vi "Arduino Drive.vi"() -> ()   [LabVIEW 2013]
panel:
  out "Back Flower Activated?":bool
  out "Right Flower Activated?":bool
  out "Intake Activated?":bool
  out "Intake -1, 1 (Suck In/Suck Out)":dbl
  out "Doggear Out/Engaged (T/F)":bool
  out "Back Flower Out/In (T/F)":bool
  out "Right Flower Out/In (T/F)":bool
  out "Intake Out/In (T/F)":bool
  in  "KeyInput":T1(ring)
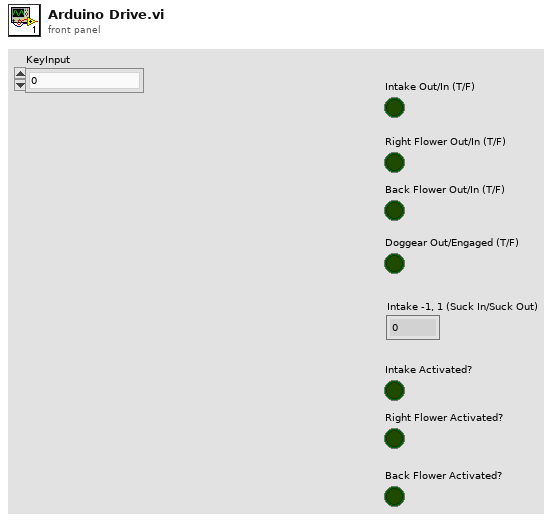
[diagram p1: front panel]
types:
  T1 = enum16{"0", "1", "2", "3", "4", "5", "6", "7", "8", "9", "A", "B", "C", "D", "E", "F", "G", "H", "I", "J", "K", "L", "M", "N", "O", "P", "Q", "R", "S", "T", "U", "V", "W", "X", "Y", "Z", "F1", "F2", "F3", "F4", "F5", "F6", "F7", "F8", "F9", "F10", "F11", "F12", "F13", "F14", "F15", "ADD", "BACK", "BACKSLASH", "CAPITAL", "COMMA", "DECIMAL", "DELETE", "DIVIDE", "DOWN", "END", "EQUALS", "ESCAPE", "GRAVE (`)", "HOME", "INSERT", "LBRACKET", "LCONTROL", "LEFT", "L ALT", "LSHIFT", "LWIN", "MINUS", "MULTIPLY", "NEXT", "NUMLOCK", "NUMPAD_0", "NUMPAD_1", "NUMPAD_2", "NUMPAD_3", "NUMPAD_4", "NUMPAD_5", "NUMPAD_6", "NUMPAD_7", "NUMPAD_8", "NUMPAD_9", "PAUSE", "PERIOD", "PRIOR (PG UP)", "RBRACKET", "RCONTROL", "RETURN", "RIGHT", "R ALT", "RSHIFT", "RWIN", "SCROLL", "SEMICOLON", "SLASH", "SPACE", "SUBTRACT", "TAB", "UP", "ENTER (num pad)", "' (quote)"}
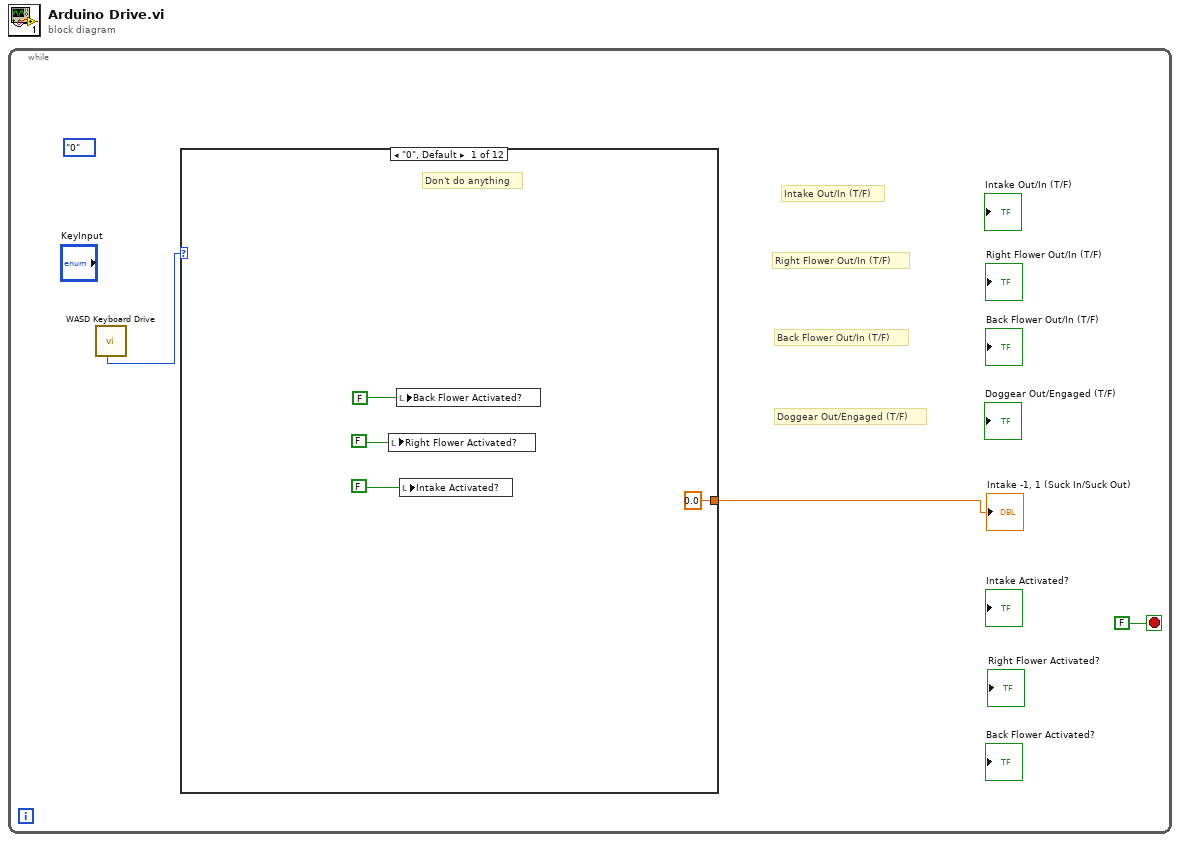
[diagram p0: block diagram]
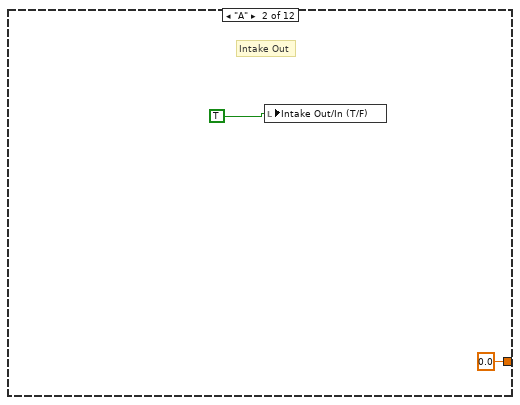
[diagram p2: hidden frame]
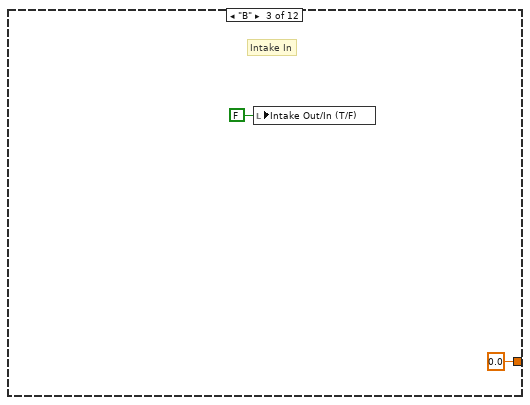
[diagram p3: hidden frame]
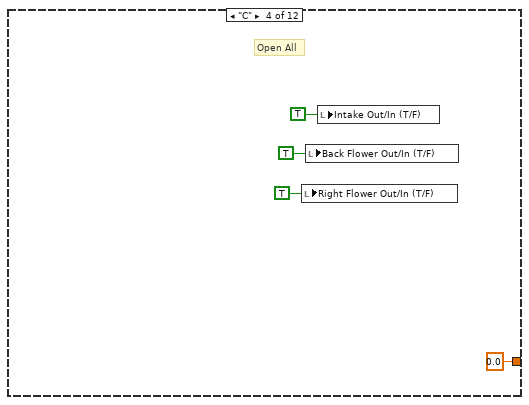
[diagram p4: hidden frame]
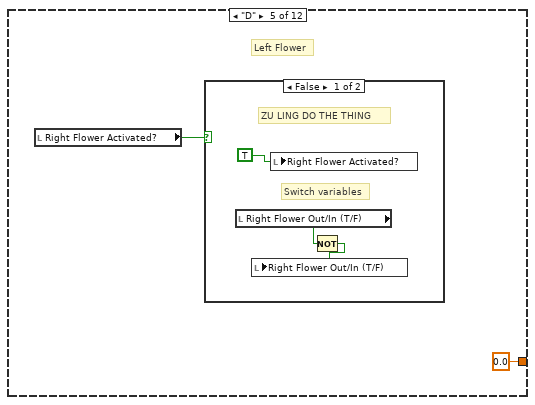
[diagram p5: hidden frame]
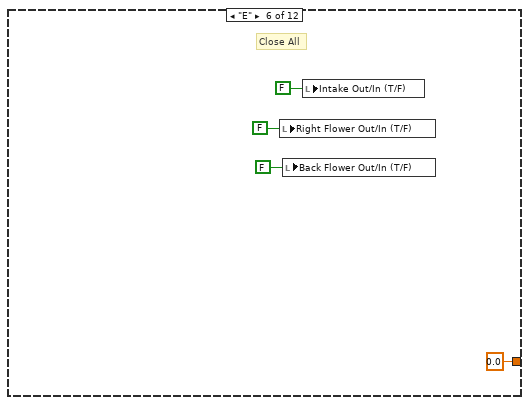
[diagram p7: hidden frame]
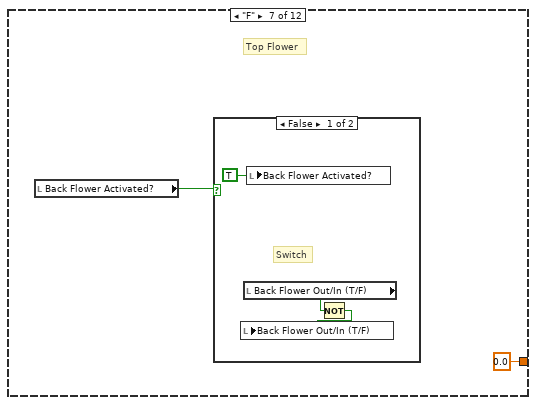
[diagram p8: hidden frame]
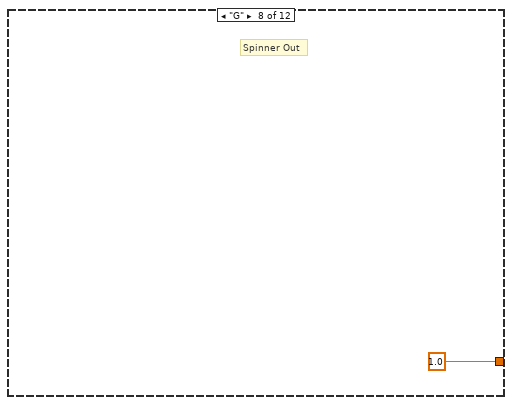
[diagram p10: hidden frame]
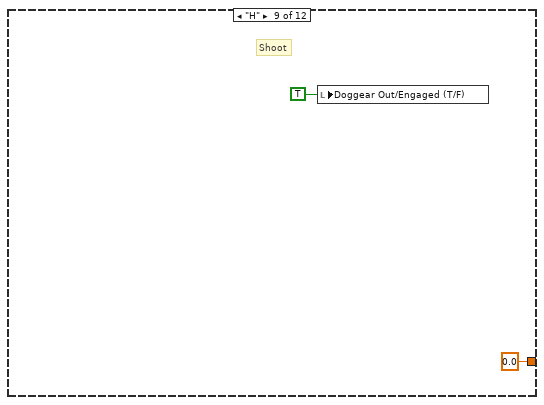
[diagram p11: hidden frame]
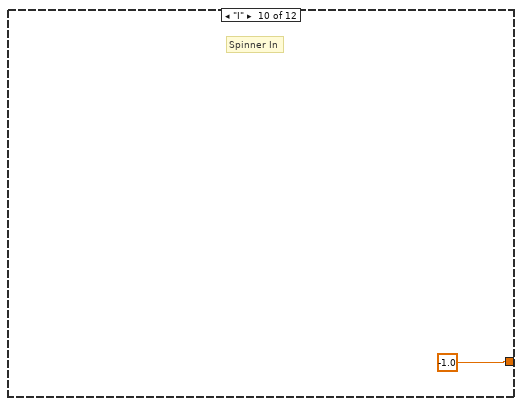
[diagram p12: hidden frame]
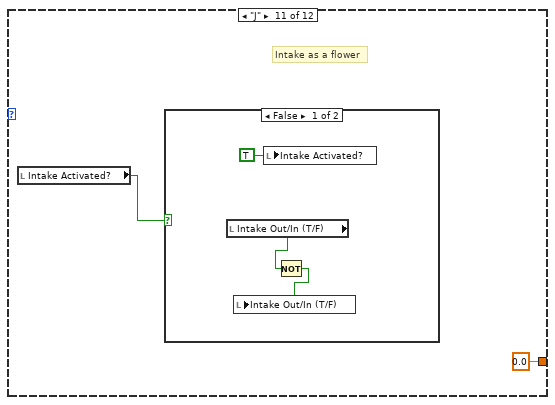
[diagram p13: hidden frame]
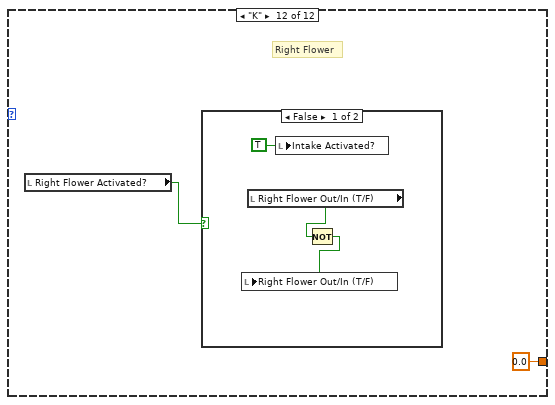
[diagram p15: hidden frame]
diagram:
  n1 = while {
    stop <- FALSE stop-if-true
    (unwired) T1."0" ("key")
    # "Doggear Out/Engaged (T/F)"
    # "Back Flower Out/In (T/F)"
    # "Right Flower Out/In (T/F)"
    # "Intake Out/In (T/F)"
    n2 = call "WASD Keyboard Drive.vi"() -> ("key"=w1:T1)  [unwired: 5 in, 2 out]
    n3 = case shown="\"0\", Default" w1 {
      tunnel: [0.0 ("Intake -1, 1 (Suck In/Suck Out)") 0.0 ("Intake -1, 1 (Suck In/Suck Out)") 0.0 ("Intake -1, 1 (Suck In/Suck Out)") 0.0 ("Intake -1, 1 (Suck In/Suck Out)") 0.0 ("Intake -1, 1 (Suck In/Suck Out)") 0.0 ("Intake -1, 1 (Suck In/Suck Out)") 0.0 ("Intake -1, 1 (Suck In/Suck Out)") 1.0 ("Intake -1, 1 (Suck In/Suck Out)") 0.0 ("Intake -1, 1 (Suck In/Suck Out)") -1.0 ("Intake -1, 1 (Suck In/Suck Out)") 0.0 ("Intake -1, 1 (Suck In/Suck Out)") 0.0 ("Intake -1, 1 (Suck In/Suck Out)")] -> w3
      frame "0", Default {
        # "Don't do anything"
        n4 = local write "Right Flower Activated?"(FALSE ("Right Flower Activated?")) -> ()
        n5 = local write "Back Flower Activated?"(FALSE ("Right Flower Activated?")) -> ()
        n6 = local write "Intake Activated?"(FALSE ("Right Flower Activated?")) -> ()
      }
      frame "A" {
        # "Intake Out"
        n7 = local write "Intake Out/In (T/F)"(TRUE) -> ()
      }
      frame "B" {
        # "Intake In"
        n8 = local write "Intake Out/In (T/F)"(FALSE ("Intake Out/In (T/F)")) -> ()
      }
      frame "C" {
        # "Open All"
        n9 = local write "Right Flower Out/In (T/F)"(TRUE ("Right Flower Out/In (T/F)")) -> ()
        n10 = local write "Back Flower Out/In (T/F)"(TRUE ("Back Flower Out/In (T/F)")) -> ()
        n11 = local write "Intake Out/In (T/F)"(TRUE ("Intake Out/In (T/F)")) -> ()
      }
      frame "D" {
        # "Left Flower"
        n12 = local read "Right Flower Activated?"() -> (w16:bool)
        n13 = case shown="False" w16 {
          frame False {
            # "Switch variables"
            # "ZU LING DO THE THING"
            n14 = local read "Right Flower Out/In (T/F)"() -> (w18:bool)
            n15 = local write "Right Flower Activated?"(TRUE) -> ()
            n16 = Not(x=w18) -> (.not. x?=w19:bool)
            n17 = local write "Right Flower Out/In (T/F)"(w19) -> ()
          }
          frame True {
            # "In a held down state"
          }
        }
      }
      frame "E" {
        # "Close All"
        n18 = local write "Right Flower Out/In (T/F)"(FALSE ("Right Flower Out/In (T/F)")) -> ()
        n19 = local write "Back Flower Out/In (T/F)"(FALSE ("Back Flower Out/In (T/F)")) -> ()
        n20 = local write "Intake Out/In (T/F)"(FALSE ("Intake Out/In (T/F)")) -> ()
      }
      frame "F" {
        # "Top Flower"
        n21 = local read "Back Flower Activated?"() -> (w25:bool)
        n22 = case shown="False" w25 {
          frame False {
            # "Switch"
            n23 = local read "Back Flower Out/In (T/F)"() -> (w28:bool)
            n24 = local write "Back Flower Activated?"(TRUE ("Back Flower Activated?")) -> ()
            n25 = Not(x=w28) -> (.not. x?=w29:bool)
            n26 = local write "Back Flower Out/In (T/F)"(w29) -> ()
          }
          frame True {
          }
        }
      }
      frame "G" {
        # "Spinner Out"
      }
      frame "H" {
        # "Shoot"
        n27 = local write "Doggear Out/Engaged (T/F)"(TRUE ("Doggear Out/Engaged (T/F)")) -> ()
      }
      frame "I" {
        # "Spinner In"
      }
      frame "J" {
        # "Intake as a flower"
        n28 = local read "Intake Activated?"() -> (w34:bool)
        n29 = case shown="False" w34 {
          frame False {
            n30 = local read "Intake Out/In (T/F)"() -> (w37:bool)
            n31 = local write "Intake Activated?"(TRUE ("Intake Activated?")) -> ()
            n32 = Not(x=w37) -> (.not. x?=w38:bool)
            n33 = local write "Intake Out/In (T/F)"(w38) -> ()
          }
          frame True {
          }
        }
      }
      frame "K" {
        # "Right Flower"
        n34 = local read "Right Flower Activated?"() -> (w39:bool)
        n35 = case shown="False" w39 {
          frame False {
            n36 = local read "Right Flower Out/In (T/F)"() -> (w42:bool)
            n37 = local write "Intake Activated?"(TRUE ("Intake Activated?")) -> ()
            n38 = Not(x=w42) -> (.not. x?=w43:bool)
            n39 = local write "Right Flower Out/In (T/F)"(w43) -> ()
          }
          frame True {
          }
        }
      }
    }
    "Intake -1, 1 (Suck In/Suck Out)" <- w3
  }
